vi "origin_test.vi"() -> ()   [LabVIEW 2013]
uses:
  <vilib>/Utility/file.llb/Read From Spreadsheet File (DBL).vi
panel:
  in  "X Long Name":string
  in  "X Units":string
  in  "Y1 Long Name":string
  in  "Y1 Units":string
  in  "Y2 Long Name":string
  in  "Y2 Units":string
  in  "Y3 Long Name":string
  in  "Y3 Units":string
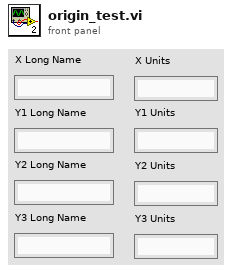
[diagram p1: front panel]
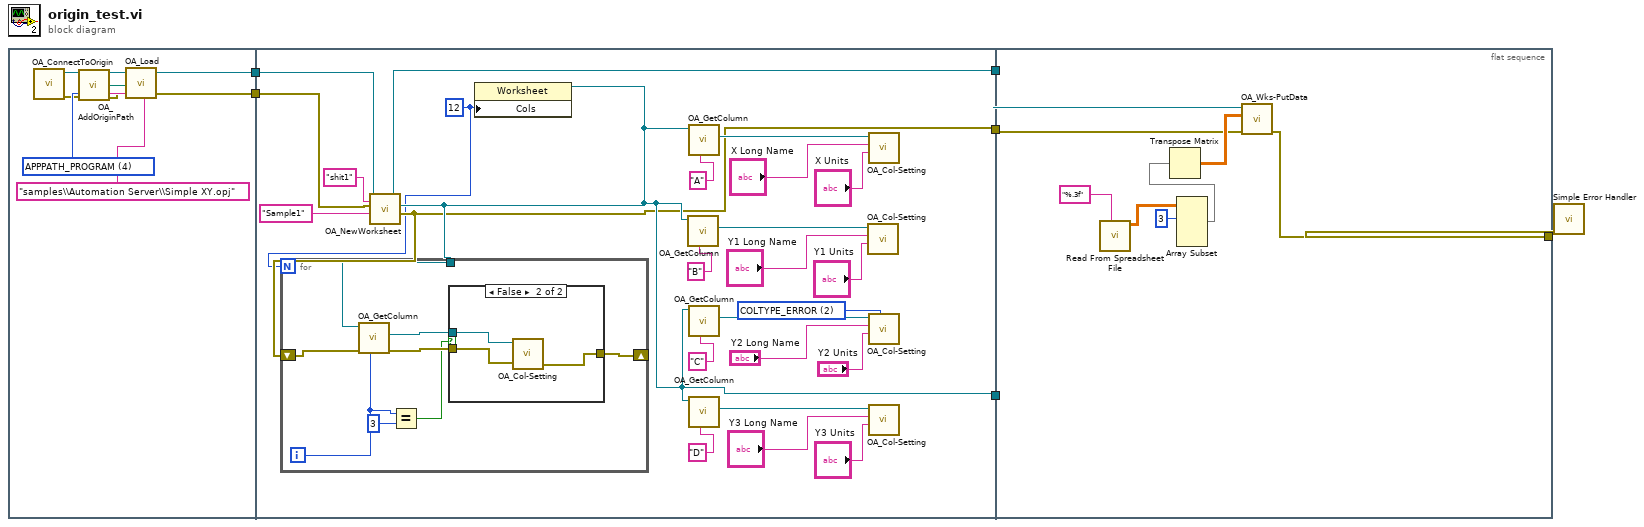
[diagram p0: block diagram]
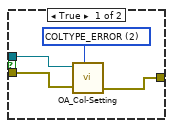
[diagram p2: hidden frame]
diagram:
  n1 = flat-sequence {
    tunnel: [w8] -> w6
    tunnel: [w7] -> w5
    tunnel: w6 -> [w23]
    tunnel: w5 -> [w24]
    tunnel: [w20] -> w4
    tunnel: [w18] -> w3
    tunnel: [w17] -> w1
    tunnel: w4 -> [_]
    tunnel: w3 -> [w63]
    tunnel: [w62] -> w2
    tunnel: w1 -> [w56]
    frame #0 {
      w13 = 4 items=["APPPATH_USER"=2, "APPPATH_GROUP"=3, "APPPATH_PROGRAM"=4] ("Type")
      n2 = call "OA_ConnectToOrigin.vi"() -> ("error out"=w9:errorcluster, "Origin.IOApplication"=w15:refnum<k7>)  [unwired: 8 in]
      n3 = call "OA_AddOriginPath.vi"("Origin.IOApplication"=w15, "error in (no error)"=w9, "Type"=w13, "Filename"="samples\\Automation Server\\Simple XY.opj" ("related path")) -> ("Origin.IOApplication"=w10:refnum<k7>, "path out"=w12:path, "error out"=w11:errorcluster)  [unwired: 9 in]
      n4 = call "OA_Load.vi"("error in (no error)"=w11, "Path"=w12, "Origin.IOApplication"=w10) -> ("error out"=w8:errorcluster, "Origin.IOApplication"=w7:refnum<k7>)  [unwired: 1 out]
    }
    frame #1 {
      w19 = 2 items=["COLTYPE_NO_CHANGE"=-1, "COLTYPE_Y"=0, "COLTYPE_NONE"=1, "COLTYPE_ERROR"=2, "COLTYPE_X"=3, "COLTYPE_LABEL"=4, "COLTYPE_Z"=5, "COLTYPE_X_ERROR"=6, "COLTYPE_GROUP"=7, "COLTYPE_SUBJECT"=8] ("Type")
      w16 = 12
      n5 = call "OA_NewWorksheet.vi"("Sheet Name"="shit1", "Book Name"="Sample1", "error in (no error)"=w23, "Origin.IOApplication"=w24) -> ("error out"=w17:errorcluster, "Origin.Worksheet"=w18:refnum<k7>, "Origin.IOApplication"=w20:refnum<k7>)  [unwired: 3 in]
      n6 = for {
        N: w16 -> [_]
        tunnel: w18 -> [w48]
        shift-right: [w45] -> _
        shift-left: w17 -> [w44]
        i -> [w43]
        n7 = call "OA_GetColumn.vi"("Column Name/Index"=w43, "error in (no error)"=w44, "Origin.Worksheet"=w48) -> ("error out"=w46:errorcluster, "Origin.Column"=w47:refnum<k7>)  [unwired: 6 in, 1 out]
        n8 = Equal?(x=w43, y=3) -> (x = y?=w41:bool)
        n9 = case shown="False" w41 {
          tunnel: w47 -> [w52 w55]
          tunnel: w46 -> [w51 w54]
          tunnel: [w50 w53] -> w45
          frame True {
            w49 = 2 items=["COLTYPE_NO_CHANGE"=-1, "COLTYPE_Y"=0, "COLTYPE_NONE"=1, "COLTYPE_ERROR"=2, "COLTYPE_X"=3, "COLTYPE_LABEL"=4, "COLTYPE_Z"=5, "COLTYPE_X_ERROR"=6, "COLTYPE_GROUP"=7, "COLTYPE_SUBJECT"=8] ("Type")
            n10 = call "OA_Col-Setting.vi"("Origin.Column"=w52, "Type"=w49, "error in (no error)"=w51) -> ("error out"=w50:errorcluster)  [unwired: 4 in, 1 out]
          }
          frame False {
            n11 = call "OA_Col-Setting.vi"("Origin.Column"=w55, "error in (no error)"=w54) -> ("error out"=w53:errorcluster)  [unwired: 5 in, 1 out]
          }
        }
      }
      n12 = property class="Worksheet"(reference=w18, "Cols"=w16) -> ()  [unwired: 1 in, 2 out]
      n13 = call "OA_GetColumn.vi"("Column Name/Index"="B" ("Name"), "Origin.Worksheet"=w18) -> ("Origin.Column"=w36:refnum<k7>)  [unwired: 7 in, 2 out]
      n14 = call "OA_GetColumn.vi"("Column Name/Index"="A" ("Name"), "Origin.Worksheet"=w18) -> ("Origin.Column"=w40:refnum<k7>)  [unwired: 7 in, 2 out]
      n15 = call "OA_GetColumn.vi"("Column Name/Index"="C" ("Name"), "Origin.Worksheet"=w18) -> ("Origin.Column"=w32:refnum<k7>)  [unwired: 7 in, 2 out]
      n16 = call "OA_GetColumn.vi"("Column Name/Index"="D" ("Name"), "Origin.Worksheet"=w18) -> ("Origin.Column"=w28:refnum<k7>)  [unwired: 7 in, 2 out]
      n17 = call "OA_Col-Setting.vi"("Origin.Column"=w36, "LongName"="Y1 Long Name", "Units"="Y1 Units") -> ()  [unwired: 4 in, 2 out]
      n18 = call "OA_Col-Setting.vi"("Origin.Column"=w40, "LongName"="X Long Name", "Units"="X Units") -> ()  [unwired: 4 in, 2 out]
      n19 = call "OA_Col-Setting.vi"("Origin.Column"=w32, "Type"=w19, "LongName"="Y2 Long Name", "Units"="Y2 Units") -> ()  [unwired: 3 in, 2 out]
      n20 = call "OA_Col-Setting.vi"("Origin.Column"=w28, "LongName"="Y3 Long Name", "Units"="Y3 Units") -> ()  [unwired: 4 in, 2 out]
    }
    frame #2 {
      n21 = call-poly <vilib>:"Read From Spreadsheet File.vi"("format (%.3f)"="%.3f") -> ("all rows"=w59:dbl[][])  [unwired: 6 in, 4 out]
      n22 = Array Subset(array=w59, index (row)=3 ("index")) -> (w57:dbl[][])  [unwired: 3 in]
      n23 = Transpose Matrix(1:w57) -> (0:w60:dbl[][])
      n24 = call "OA_Wks-PutData.vi"("error in (no error)"=w56, "2d Data"=w60, "Origin.Worksheet"=w63) -> ("error out"=w62:errorcluster)  [unwired: 2 in, 2 out]
    }
  }
  n25 = call <vilib>:"Simple Error Handler.vi"("error in (no error)"=w2) -> ()  [unwired: 4 in, 5 out]
